vi "check_timeout.vi"(8 "error in (no error)":errorcluster, 11 "Experiment (in)":refnum<class "Experiment.lvclass">) -> (0 "error out":errorcluster, 2 "timeout elapsed?":bool, 3 "Experiment":refnum<class "Experiment.lvclass">)   [LabVIEW 2013, in "Experiment.lvclass"]
uses:
  Experiment.lvclass
  Experiment.lvclass/Experiment.ctl
  Globals.vi
panel:
  out "millisecond timer value":u32
  out "Timeout Elapses At":u32
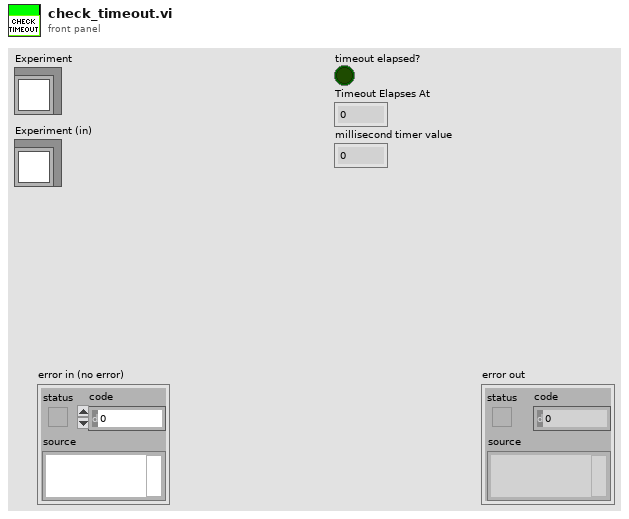
[diagram p1: front panel]
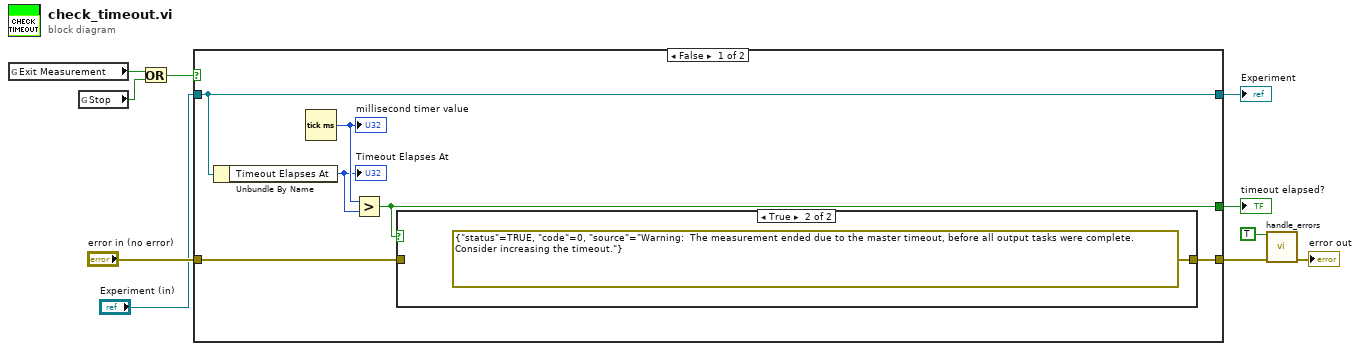
[diagram p0: block diagram]
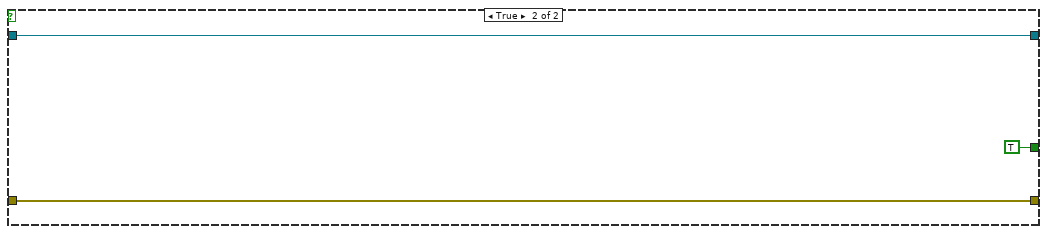
[diagram p3: hidden frame]
diagram:
  n1 = global read "Globals.vi" "Exit Measurement"() -> (w8:bool)
  n2 = global read "Globals.vi" "Stop"() -> (w7:bool)
  n3 = Or(x=w8, y=w7) -> (x .or. y?=w6:bool)
  n4 = case shown="False" w6 {
    tunnel: [w13 w20] -> w2
    tunnel: [w16 w21] -> w4
    tunnel: "Experiment (in)" -> [w16 w21]
    tunnel: [w12 TRUE] -> w10
    tunnel: "error in (no error)" -> [w11 w20]
    frame False {
      n5 = Unbundle By Name(w16) -> ("Timeout Elapses At"=w14:u32)
      "Timeout Elapses At" <- w14
      n6 = Tick Count (ms)() -> (millisecond timer value=w15:u32)
      "millisecond timer value" <- w15
      n7 = Greater?(x=w15, y=w14) -> (0:w12:bool)
      n8 = case shown="True" w12 {
        tunnel: [w17 errorcluster {"status"=TRUE, "code"=0, "source"="Warning:  The measurement ended due to the master timeout, before all output tasks were complete.  Consider increasing the timeout."} ("error constant")] -> w13
        tunnel: w11 -> [w17 _]
        frame False {
        }
        frame True {
        }
      }
    }
    frame True {
    }
  }
  "timeout elapsed?" <- w10
  "Experiment" <- w4
  n9 = call "handle_errors.vi"("Exit Operation"=TRUE ("Exit Measurement"), "error in (no error)"=w2) -> ("error out"=→"error out":errorcluster)  [unwired: 13 in]
